vi "csm_lumikki_instron_moveToSetpoint.vi"(10 "setPointTime":dbl=1.0, 11 "setPoint":dbl=1.0) -> (2 "setpointTimeOut":dbl, 3 "setpointOut":dbl, 6 "newSetpointCommand":bool)   [LabVIEW 2009]
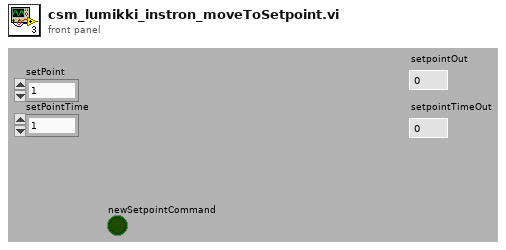
[diagram p1: front panel]
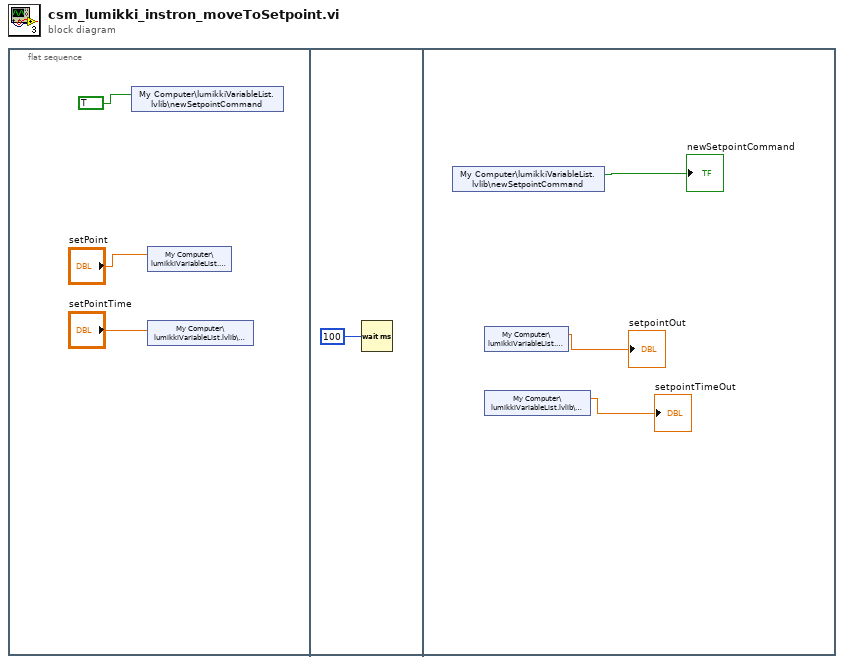
[diagram p0: block diagram]
diagram:
  n1 = flat-sequence {
    frame #0 {
      n2 = shared-variable "My Computer\\lumikkiVariableList.lvlib\\newSetpointCommand"(TRUE ("Busy")) -> ()  [unwired: 1 in, 1 out]
      n3 = shared-variable "My Computer\\lumikkiVariableList.lvlib\\setpoint"("setPoint") -> ()  [unwired: 1 in, 1 out]
      n4 = shared-variable "My Computer\\lumikkiVariableList.lvlib\\setpointTime"("setPointTime") -> ()  [unwired: 1 in, 1 out]
    }
    frame #1 {
      n5 = Wait (ms)(milliseconds to wait=u32 100) -> ()  [unwired: 1 out]
    }
    frame #2 {
      n6 = shared-variable "My Computer\\lumikkiVariableList.lvlib\\newSetpointCommand"() -> (→"newSetpointCommand":bool)  [unwired: 1 in, 1 out]
      n7 = shared-variable "My Computer\\lumikkiVariableList.lvlib\\setpoint"() -> (→"setpointOut":dbl)  [unwired: 1 in, 1 out]
      n8 = shared-variable "My Computer\\lumikkiVariableList.lvlib\\setpointTime"() -> (→"setpointTimeOut":dbl)  [unwired: 1 in, 1 out]
    }
  }
